vi "Get git branch name.vi"(2 "git branch name":string, 8 "error in (no error)":errorcluster, 11 "FPGA Interface in":refnum<class "FPGA Interface.lvclass">) -> (0 "error out":errorcluster, 3 "FPGA Interface out":refnum<class "FPGA Interface.lvclass">)   [LabVIEW 2026, in "TALOS.lvlib" / "Interfaces.lvlib" / "FPGA Interface.lvclass"]
uses:
  FPGA Interface.lvclass
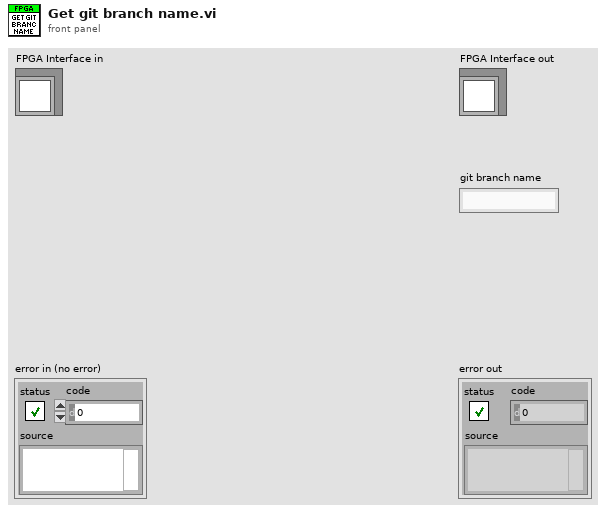
[diagram p1: front panel]
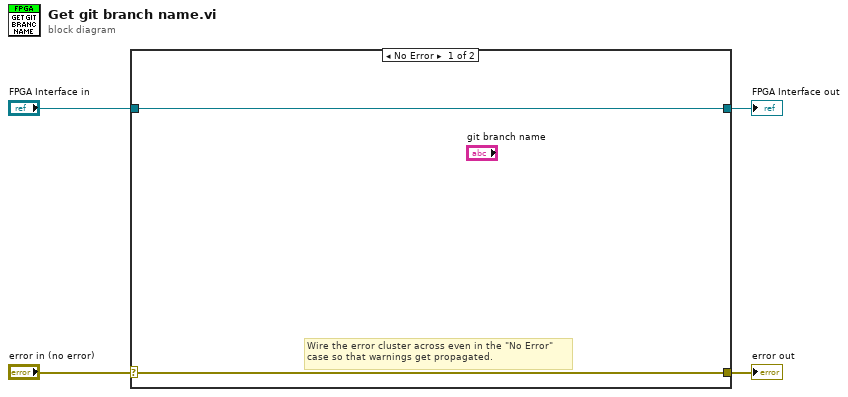
[diagram p0: block diagram]
diagram:
  n1 = case shown="No Error" "error in (no error)" {
    selector: "error in (no error)" -> [w5 w8]
    tunnel: [w5 w8] -> w3
    tunnel: [w6 w7] -> w1
    tunnel: "FPGA Interface in" -> [w6 w7]
    frame No Error {
      # "Wire the error cluster across even in the \"No Error\"\ncase so that warnings get propagated."
    }
    frame Error {
    }
  }
  "error out" <- w3
  "FPGA Interface out" <- w1
